vi "Write Data.vi"(8 "error in (no error)":errorcluster, 10 "Data":i32, 11 "RequestStatus Msg in":refnum<class "RequestStatus Msg.lvclass">) -> (0 "error out":errorcluster, 3 "RequestStatus Msg out":refnum<class "RequestStatus Msg.lvclass">)   [LabVIEW 2016, in "MyBaseActor.lvlib" / "RequestStatus Msg.lvclass"]
uses:
  RequestStatus Msg.lvclass
  RequestStatus Msg.lvclass/RequestStatus Msg.ctl
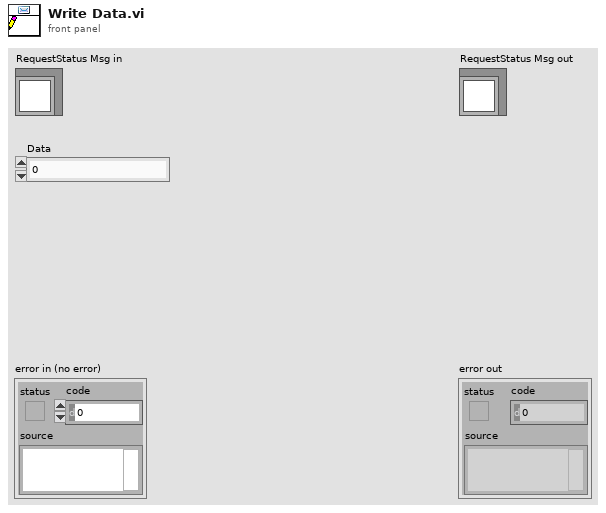
[diagram p1: front panel]
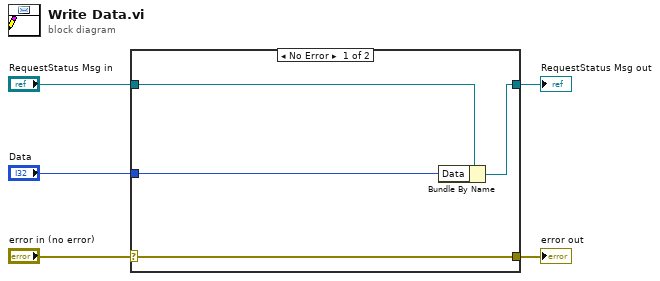
[diagram p0: block diagram]
diagram:
  n1 = case shown="No Error" "error in (no error)" {
    selector: "error in (no error)" -> [w9 w10]
    tunnel: [w9 w10] -> w4
    tunnel: [w7 w11] -> w2
    tunnel: "RequestStatus Msg in" -> [w8 w11]
    tunnel: "Data" -> [w6 _]
    frame No Error {
      n2 = Bundle By Name(cluster=w8, "Data"=w6) -> (w7:refnum<class "RequestStatus Msg.lvclass">)
    }
    frame Error {
    }
  }
  "error out" <- w4
  "RequestStatus Msg out" <- w2
